vi "연속쓰기요구(subVI).vi"(1 "데이터":u16[](array[numeric])=[13106, 13104, 13107, 13108, 9521, 12848, 13620, 13879] format="%.0x", 2 "직접변수":string="%DB0000") -> (0 "연속쓰기":string)   [LabVIEW 2014]
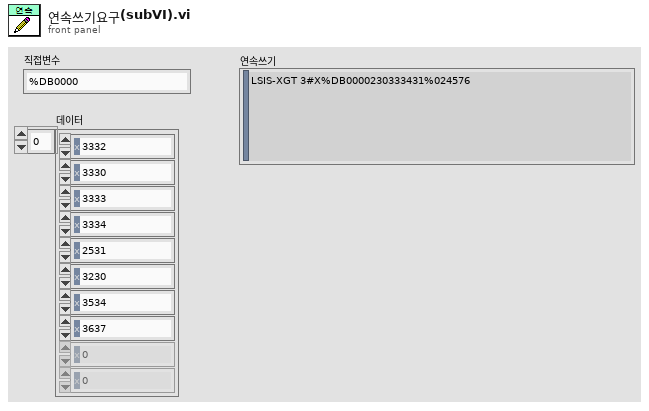
[diagram p1: front panel]
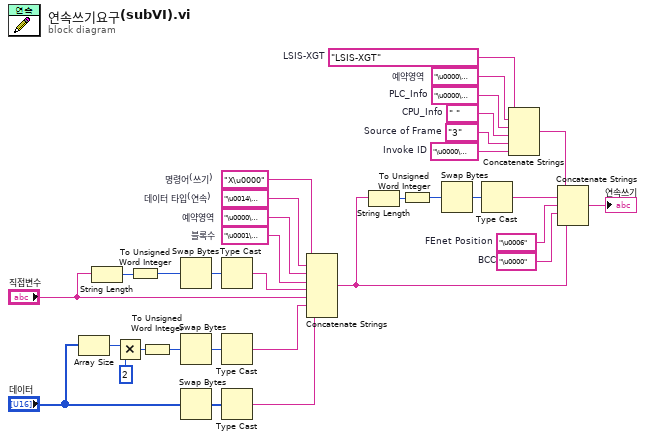
[diagram p0: block diagram]
diagram:
  w20 = "\u0001\u0000"  # 블록수
  w22 = "\u0000"  # BCC
  w23 = "\u0006"  # FEnet Position
  w25 = "\u0000\u0000"  # Invoke ID
  w26 = "3"  # Source of Frame
  w27 = " "  # CPU_Info
  w28 = "\u0000\u0000"  # PLC_Info
  w29 = "\u0000\u0000"  # 예약영역
  w30 = "LSIS-XGT"  # LSIS-XGT
  w2 = "\u0000\u0000"  # 예약영역
  w32 = "\u0014\u0000"  # 데이터 타입(연속)
  w33 = "X\u0000"  # 명령어(쓰기)
  n1 = Array Size(array="데이터") -> (size(s)=w11:i32)
  n2 = String Length(string="직접변수") -> (length=w19:i32)
  n3 = Multiply(x=w11, y=2) -> (x*y=w10:i32)
  n4 = To Unsigned Word Integer(number=w19) -> (unsigned 16bit integer=w18:u16)
  n5 = To Unsigned Word Integer(number=w10) -> (unsigned 16bit integer=w13:u16)
  n6 = Swap Bytes(anything=w18) -> (byte swapped=w17:u16)
  n7 = Swap Bytes(anything=w13) -> (byte swapped=w14:u16)
  n8 = Swap Bytes(anything="데이터") -> (byte swapped=w8:u16[])
  n9 = Type Cast(x=w17) -> (*(type *) &x=w16:string)  [unwired: 1 in]
  n10 = Type Cast(x=w14) -> (*(type *) &x=w12:string)  [unwired: 1 in]
  n11 = Type Cast(x=w8) -> (*(type *) &x=w7:string)  [unwired: 1 in]
  n12 = Concatenate Strings(w33, w32, w2, w20, w16, "직접변수", w12, w7) -> (w24:string)
  n13 = String Length(string=w24) -> (length=w31:i32)
  n14 = To Unsigned Word Integer(number=w31) -> (unsigned 16bit integer=w6:u16)
  n15 = Swap Bytes(anything=w6) -> (byte swapped=w5:u16)
  n16 = Type Cast(x=w5) -> (*(type *) &x=w4:string)  [unwired: 1 in]
  n17 = Concatenate Strings(w30, w29, w28, w27, w26, w25) -> (w3:string)
  n18 = Concatenate Strings(w3, w4, w23, w22, w24) -> (→"연속쓰기":string)
